vi "receiver.vi"() -> ()   [LabVIEW 2013]
uses:
  <vilib>/sound2/lvsound2.llb/Sound Data Format.ctl
  <vilib>/sound2/lvsound2.llb/Sampling Mode.ctl
  Receiver/Receiver.lvclass
  <vilib>/sound2/lvsound2.llb/Sound Input Read (DBL).vi
panel:
  out "string":string
  out "Array":i32[](array[numeric])
  in  "stop":bool
  in  "Duration (s)":dbl=0.05
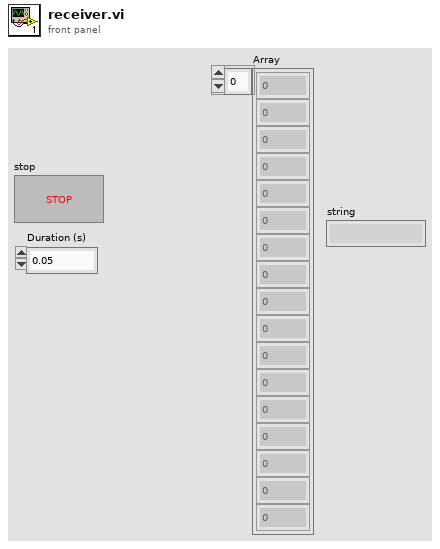
[diagram p1: front panel]
types:
  T1 = typedef "Sampling Mode.ctl" = i32
  T2 = typedef "Sound Data Format.ctl" = cluster{"sample rate (S/s)":dbl, "number of channels":i32, "bits per sample":i32}
  T3 = typedef "Sound Input Task ID.ctl" = u32
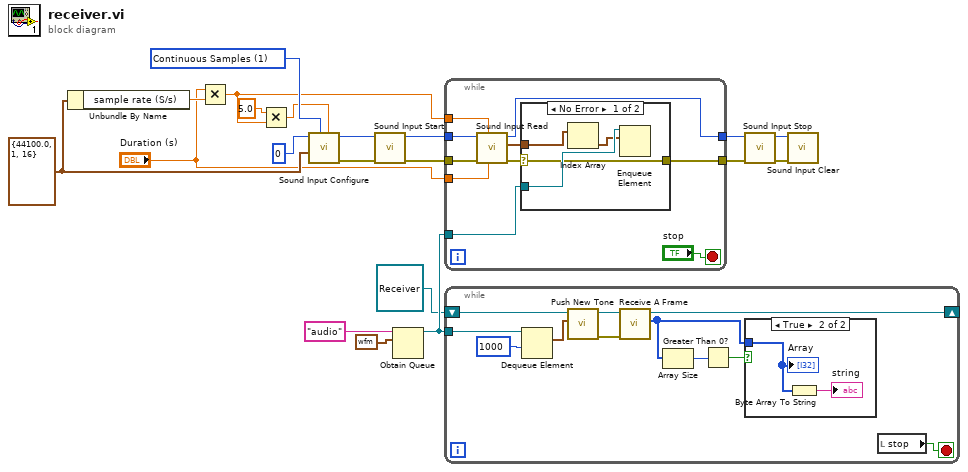
[diagram p0: block diagram]
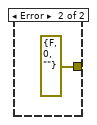
[diagram p3: hidden frame]
diagram:
  w20 = T1 1 items=["Finite Samples", "Continuous Samples"] ("sample mode")
  w18 = T2 {"sample rate (S/s)"=44100.0, "number of channels"=1, "bits per sample"=16} ("sound format")
  n1 = Unbundle By Name(w18) -> ("sample rate (S/s)"=w17:dbl)
  n2 = Multiply(x="Duration (s)", y=w17) -> (x*y=w13:dbl)
  n3 = Multiply(x=5.0, y=w13) -> (x*y=w3:dbl)
  n4 = call <vilib>:"Sound Input Configure.vi"("number of samples/ch"=w3, "sample mode"=w20, "sound format"=w18, "device ID"=u32 0) -> ("error out"=w15:errorcluster, "task ID"=w16:T3)  [unwired: 6 in]
  n5 = call <vilib>:"Sound Input Start.vi"("error in (no error)"=w15, "task ID"=w16) -> ("error out"=w10:errorcluster, "task ID out"=w14:T3)  [unwired: 8 in]
  n6 = Obtain Queue(name (unnamed)="audio", element data type=waveform(dbl) {"t0"=timestamp(0 s since 1904-01-01), "dt"=1.0, "Y"=[]} ("element")) -> (queue out=w6:refnum<queue>)  [unwired: 3 in, 2 out]
  n7 = while {
    tunnel: w14 -> [w29]
    tunnel: w13 -> [w28]
    tunnel: [w27] -> w11
    tunnel: w10 -> [w26]
    tunnel: [w21] -> w9
    tunnel: w6 -> [w24]
    tunnel: "Duration (s)" -> [w23]
    stop <- "stop" stop-if-true
    n8 = call-poly <vilib>:"Sound Input Read.vi"("timeout (sec)"=w23, "number of samples/ch"=w28, "error in (no error)"=w26, "task ID"=w29) -> ("error out"=w22:errorcluster, "data"=w25:waveform(dbl)[], "task ID out"=w27:T3)  [unwired: 5 in]
    n9 = case shown="No Error" w22 {
      selector: w22 -> [w31 _]
      tunnel: w25 -> [w34 _]
      tunnel: w24 -> [w33 _]
      tunnel: [w31 errorcluster {"status"=FALSE, "code"=0, "source"=""} ("error IO")] -> w21
      frame No Error {
        n10 = Index Array(array=w34) -> (element=w32:waveform(dbl))  [unwired: 1 in]
        n11 = Enqueue Element(queue=w33, element=w32) -> ()  [unwired: 2 in, 3 out]
      }
      frame Error {
      }
    }
  }
  n12 = while {
    tunnel: w6 -> [w45]
    shift-right: [w39] -> _
    shift-left: refnum<class "Receiver.lvclass"> refnum ("Receiver.lvclass") -> [w43]
    stop <- w46 stop-if-true
    n13 = Dequeue Element(queue=w45, timeout in ms (-1)=1000) -> (element=w42:waveform(dbl))  [unwired: 1 in, 3 out]
    n14 = call-dynamic "Push New Tone.vi"("signal"=w42, "Receiver in"=w43) -> ("error out"=w40:errorcluster, "Receiver out"=w41:refnum<class "Receiver.lvclass">)  [unwired: 8 in]
    n15 = call-dynamic "Receive A Frame.vi"("error in (no error)"=w40, "Receiver in"=w41) -> ("Received data"=w38:i32[], "Receiver out"=w39:refnum<class "Receiver.lvclass">)  [unwired: 7 in, 1 out]
    n16 = Array Size(array=w38) -> (size(s)=w37:i32)
    n17 = Greater Than 0?(x=w37) -> (x > 0?=w36:bool)
    n18 = case shown="True" w36 {
      tunnel: w38 -> [_ w48]
      frame False {
      }
      frame True {
        n19 = Byte Array To String(unsigned byte array=w48) -> (string=→"string":string)
        "Array" <- w48
      }
    }
    n20 = local read "stop"() -> (w46:bool)
  }
  n21 = call <vilib>:"Sound Input Stop.vi"("error in (no error)"=w9, "task ID"=w11) -> ("error out"=w8:errorcluster, "task ID out"=w12:T3)  [unwired: 8 in]
  n22 = call <vilib>:"Sound Input Clear.vi"("error in (no error)"=w8, "task ID"=w12) -> ()  [unwired: 9 in, 1 out]
